vi "AVQ8347 Measure.vi"(8 "Error In":errorcluster, 10 "Measure Select":enum16{"Stop", "Single", "Repeat"}(ring), 11 "VISA Session":refnum<visa-resource-name>) -> (0 "Error Out":errorcluster, 2 "Send Code":string, 3 "Copy VISA Session":refnum<visa-resource-name>)   [LabVIEW 2020]
doc: "Measuring"
panel:
  # "Measure"
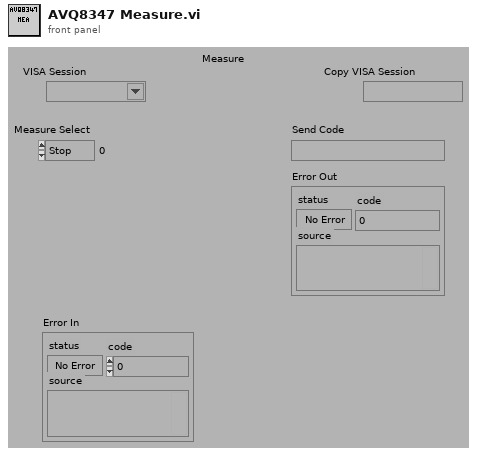
[diagram p1: front panel]
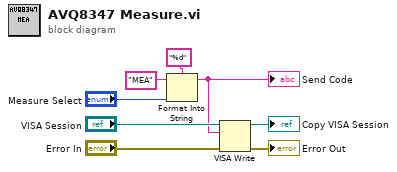
[diagram p0: block diagram]
diagram:
  n1 = Format Into String(format string="%d", initial string="MEA", "Measure Select") -> (resulting string=w1:string)  [unwired: 1 in, 1 out]
  "Send Code" <- w1
  n2 = VISA Write(VISA resource name="VISA Session", write buffer=w1, error in (no error)="Error In") -> (VISA resource name out=→"Copy VISA Session":refnum<visa-resource-name>, error out=→"Error Out":errorcluster)  [unwired: 1 out]
